vi "FlatSequence.vi"() -> ()   [LabVIEW 2019]
panel:
  in  "stop 2":bool
  out "Numeric 2":i32
  out "Numeric":i32
  in  "stop":bool
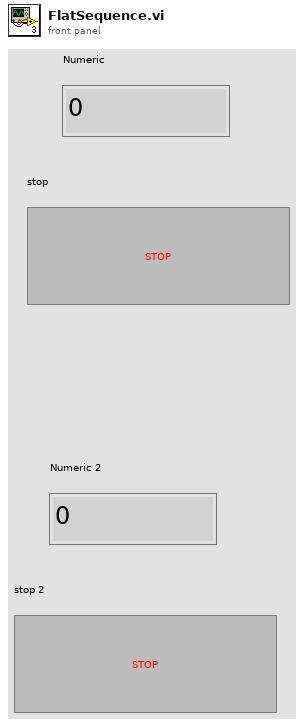
[diagram p1: front panel]
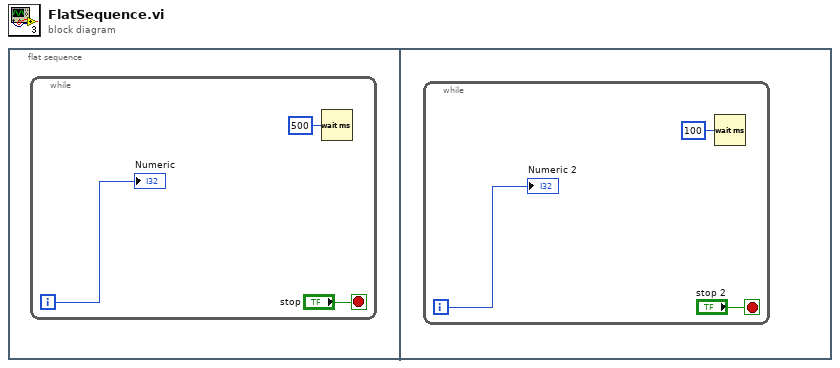
[diagram p0: block diagram]
diagram:
  n1 = flat-sequence {
    frame #0 {
      n2 = while {
        i -> [w1]
        stop <- "stop" stop-if-true
        n3 = Wait (ms)(milliseconds to wait=u32 500) -> ()  [unwired: 1 out]
        "Numeric" <- w1
      }
    }
    frame #1 {
      n4 = while {
        i -> [w4]
        stop <- "stop 2" stop-if-true
        n5 = Wait (ms)(milliseconds to wait=u32 100) -> ()  [unwired: 1 out]
        "Numeric 2" <- w4
      }
    }
  }
